vi "New Image (Greyscale Array).vi"(8 "error in (no error)":errorcluster, 11 "Greyscale Pixels (Default: Empty)":u8[][](array[numeric])) -> (0 "error out":errorcluster, 3 "Greyscale Image":T1)   [LabVIEW 2020, in "g_ar_toolkit.image.lvlib"]
uses:
  g_ar_toolkit.image.lvlib
  Greyscale Image.ctl
  g_ar_toolkit.common/g_ar_toolkit.common.lvlib
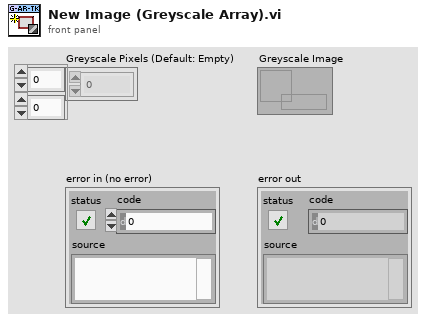
[diagram p1: front panel]
types:
  T1 = typedef "g_ar_toolkit.image.lvlib/Greyscale Image.ctl" = refnum<data-value>
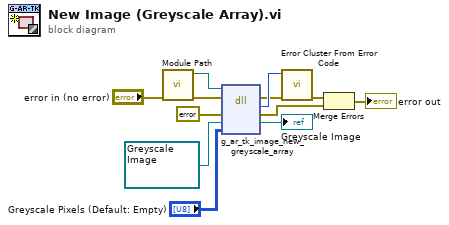
[diagram p0: block diagram]
diagram:
  n1 = call "Module Path.vi"("error in (no error)"="error in (no error)") -> ("error out"=w3:errorcluster, "Path"=w2:path)  [unwired: 9 in]
  n2 = dll-call lib="?" fn="g_ar_tk_image_new_greyscale_array" ("g_ar_toolkit.*.*:g_ar_tk_image_create")(path in=w2, error in=w3, "error_cluster"=errorcluster {"status"=FALSE, "code"=0, "source"=""} ("error constant"), "EDVR"=T1 refnum ("Ref Type"), "array_handle"="Greyscale Pixels (Default: Empty)") -> (error out=w5:errorcluster, "MgErr"=w6:i32, "error_cluster"=w12:errorcluster, "EDVR"=→"Greyscale Image":T1)  [unwired: 2 in, 1 out]
  n3 = call <vilib>:"Error Cluster From Error Code.vi"("error in (no error)"=w5, "error code (0)"=w6) -> ("error out"=w8:errorcluster)  [unwired: 7 in]
  n4 = Merge Errors(w8, w12) -> (→"error out":errorcluster)
